vi "Display.vi"(8 "error in":errorcluster, 11 "Timeout One Button in":refnum<class "Custom - Timeout One Button.lvclass">) -> (0 "error out":errorcluster, 3 "Timeout One Button out":refnum<class "Custom - Timeout One Button.lvclass">)   [LabVIEW 2021, in "Pop-Up.lvlib" / "Custom - Timeout One Button.lvclass"]
doc: "This vi displays the custom image one button timeout popup.\n\n<b>Code Developed By:</b> +\nDaniel Coons +\nhttps://github.com/danielcoons/tsc-pop-up"
uses:
  Custom - Timeout One Button.lvclass
  C:/Development/Open Source/tsc-pop-up/Popup/Popup.lvclass
  Custom - Timeout One Button.lvclass/Custom - Timeout One Button.ctl
  Popup/Popup.lvclass/Popup.ctl
  Popup/Data Member Access/Read Theme.vi
  Theme/Theme.lvclass
  Popup/Popup.lvclass
  user32.dll
panel:
  out "header":bool
  out "count":string
  in  "OK":bool
  out "Message":string
  out "2D Picture":picture
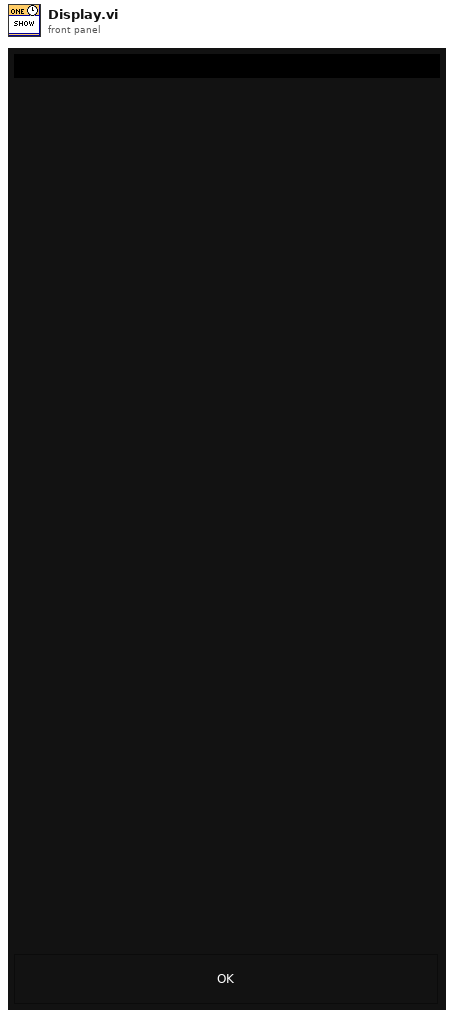
[diagram p1: front panel]
types:
  T1 = typedef "LVPoint32TypeDef.ctl" = cluster{"Horizontal":i32, "Vertical":i32}
  T2 = typedef "LVPositionTypeDef.ctl" = cluster{"Left":i32, "Top":i32}
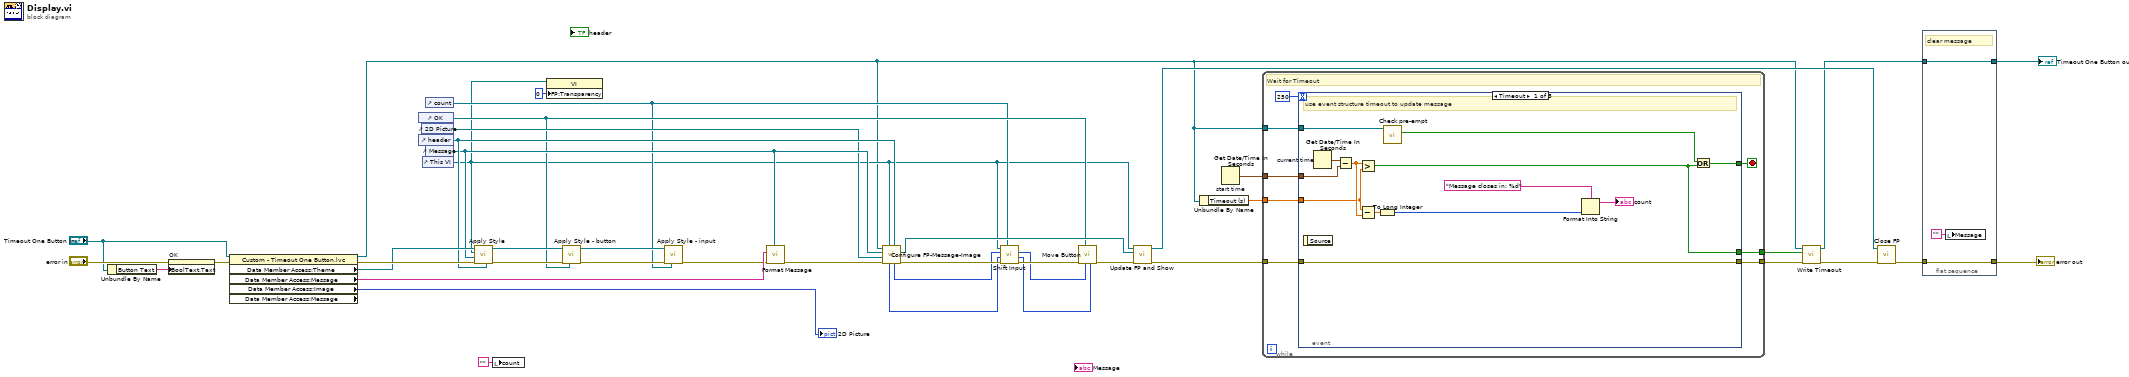
[diagram p0: block diagram]
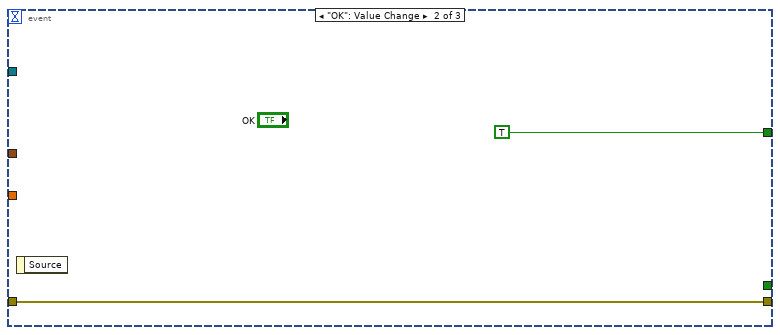
[diagram p2: hidden frame]
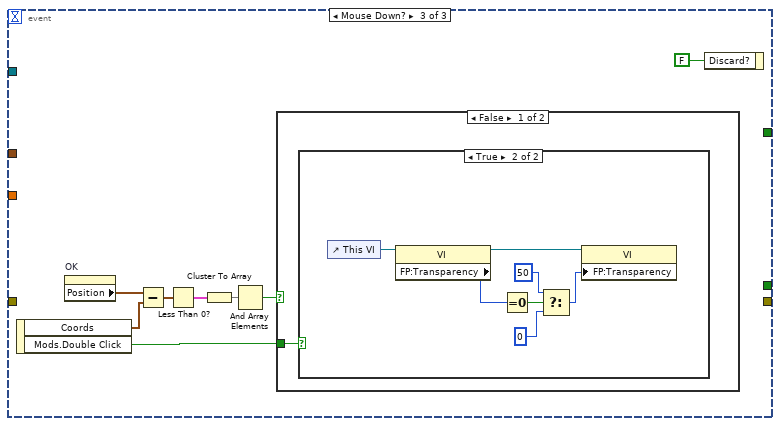
[diagram p3: hidden frame]
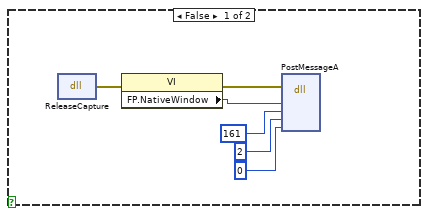
[diagram p4: hidden frame]
diagram:
  n1 = Unbundle By Name("Timeout One Button in") -> ("Button Text"=w38:string)
  n2 = property on="OK" class="Bool"(error in="error in", "BoolText.Text"=w38) -> (error out=w40:errorcluster)  [unwired: 1 in, 1 out]
  n3 = property on="Property Node" class="Custom - Timeout One Button.lvc" props=["Data Member Access:Theme", "Data Member Access:Message", "Data Member Access:Image", "Data Member Access:Message"](reference="Timeout One Button in", error in=w40) -> (reference out=w1:refnum<class "Custom - Timeout One Button.lvclass">, error out=w26:errorcluster, "Data Member Access:Theme"=w25:refnum<class "Theme.lvclass">, "Data Member Access:Message"=w23:string, "Data Member Access:Image"=→"2D Picture":picture)  [unwired: 1 out]
  n4 = control-ref of="OK"() -> (w16:refnum<vi>)
  n5 = control-ref of="header"() -> (w21:refnum<vi>)
  n6 = control-ref of="2D Picture"() -> (w19:refnum<vi>)
  n7 = control-ref of="This VI"() -> (w6:refnum<vi>)
  n8 = control-ref of="count"() -> (w11:refnum<vi>)
  n9 = control-ref of="Message"() -> (w20:refnum<vi>)
  n10 = call "Apply Style.vi"("header ref"=w21, "error in"=w26, "message ref"=w20, "pop up ref"=w6, "Theme in"=w25) -> ("error out"=w28:errorcluster, "Theme out"=w27:refnum<class "Theme.lvclass">)  [unwired: 5 in]
  n11 = local write "count"("" ("count")) -> ()
  n12 = property on="Property Node" class="VI"(reference=w6, "FP:Transparency"=u8 0 ("Front Panel Window:Transparency")) -> ()  [unwired: 1 in, 2 out]
  n13 = call "Apply Style - button.vi"("button ref"=w16, "error in"=w28, "Theme in"=w27) -> ("error out"=w24:errorcluster, "Theme out"=w13:refnum<class "Theme.lvclass">)  [unwired: 7 in]
  n14 = call "Apply Style - input.vi"("input ref"=w11, "error in (no error)"=w24, "Theme in"=w13) -> ("error out"=w14:errorcluster)  [unwired: 7 in, 1 out]
  n15 = call "Format Message.vi"("formatted string"=w20, "error in"=w14, "String Input"=w23) -> ("error out"=w22:errorcluster)  [unwired: 7 in, 1 out]
  n16 = call "Configure FP-Message-Image.vi"("header ref"=w21, "Pop Up ref"=w6, "error in (no error)"=w22, "Image ref"=w19, "Message ref"=w20, "Popup in"=w1) -> ("error out"=w18:errorcluster, "Panel Ref"=w17:refnum<vi>, "Panel Width"=w10:i32, "Panel Height"=w8:i32)  [unwired: 1 in, 1 out]
  n17 = call "Shift Input.vi"("Control"=w11, "Error In"=w18, "Panel Height"=w8, "Panel Width"=w10, "Pop Up ref"=w6) -> ("Error Out"=w12:errorcluster, "Panel Height out"=w7:i32, "Panel Width out"=w9:i32)  [unwired: 4 in]
  n18 = call "Move Button.vi"("Panel Height"=w7, "Panel Width"=w9, "Button"=w16, "error in"=w12) -> ("error out"=w15:errorcluster)  [unwired: 6 in, 1 out]
  n19 = call "Update FP and Show.vi"("error in (no error)"=w15, "Panel Ref"=w17, "VI in"=w6) -> ("error out"=w36:errorcluster, "VI out"=w32:refnum<vi>)  [unwired: 7 in]
  n20 = Unbundle By Name(w1) -> ("Timeout (s)"=w31:dbl)
  n21 = Get Date/Time In Seconds "start time"() -> (seconds since 1Jan1904=w30:timestamp)
  n22 = while {
    tunnel: [w45] -> w37
    tunnel: w36 -> [w46]
    tunnel: w30 -> [w50]
    tunnel: w31 -> [w48]
    tunnel: w1 -> [w44]
    tunnel: [w43] -> w2
    stop <- w49 stop-if-true
    # "Wait for Timeout"
    n23 = event shown="[0] Timeout" {
      selector: _ -> [_ _ _]
      dyn-events: _ -> [_ _ _]
      timeout: 250 -> [_ _ _]
      tunnel: w50 -> [w63 _ _]
      tunnel: [w54 TRUE _] -> w49
      tunnel: w48 -> [w59 _ _]
      tunnel: w46 -> [w56 w64 _]
      tunnel: [w56 w64 _] -> w45
      tunnel: w44 -> [w55 _ _]
      tunnel: [w51 _ _] -> w43
      event Timeout {
        # "use event structure timeout to update message"
        n24 = event-data() -> ()  [unwired: 1 in, 1 out]
        n25 = Get Date/Time In Seconds "current time"() -> (seconds since 1Jan1904=w62:timestamp)
        n26 = Subtract(x=w62, y=w63) -> (x-y=w61:dbl)
        n27 = Greater?(x=w61, y=w59) -> (0:w51:bool)
        n28 = Subtract(x=w59, y=w61) -> (x-y=w60:dbl)
        n29 = To Long Integer(number=w60) -> (32bit integer=w57:i32)
        n30 = call "Check pre-empt.vi"("_Popup in"=w55) -> ("Pre-empted?"=w53:bool)  [unwired: 8 in, 2 out]
        n31 = Format Into String(format string="Message closes in: %d", w57) -> (resulting string=→"count":string)  [unwired: 2 in, 1 out]
        n32 = Or(x=w53, y=w51) -> (x .or. y?=w54:bool)
      }
      event "OK": Value Change {
        n33 = event-data() -> ()  [unwired: 1 in, 1 out]
      }
      event Mouse Down? {
        n34 = event-data() -> ("Coords"=w66:T1, "Mods.Double Click"=w67:bool)  [unwired: 1 in]
        n35 = property on="OK" class="Bool"() -> ("Position"=w72:T2)  [unwired: 2 in, 2 out]
        n36 = Subtract(x=w72, y=w66) -> (x-y=w71:T2)
        n37 = Less Than 0?(x=w71) -> (x < 0?=w70:cluster{"Left":bool, "Top":bool})
        n38 = Cluster To Array(cluster=w70) -> (array=w69:bool[])
        n39 = And Array Elements(Boolean array=w69) -> (logical AND=w68:bool)
        n40 = case shown="False" w68 {
          tunnel: w67 -> [w74 _]
          frame False {
            n41 = case shown="True" w74 {
              frame False {
                n42 = dll-call lib="user32.dll" fn="ReleaseCapture"() -> (error out=w78:errorcluster)  [unwired: 4 in, 1 out]
                n43 = property on="Property Node" class="VI"(error in=w78) -> (error out=w79:errorcluster, "FP.NativeWindow"=w80:u64)  [unwired: 1 in, 1 out]
                n44 = dll-call lib="user32.dll" fn="PostMessageA"(error in=w79, "hWnd"=w80, "Msg"=161, "wParam"=2, "lParam"=0) -> ()  [unwired: 7 in, 2 out]
              }
              frame True {
                n45 = control-ref of="This VI"() -> (w87:refnum<vi>)
                n46 = property on="Property Node" class="VI"(reference=w87) -> (reference out=w85:refnum<vi>, "FP:Transparency"=w86:u8)  [unwired: 1 in, 1 out]
                n47 = Equal To 0?(x=w86) -> (x = 0?=w84:bool)
                n48 = Select(t=u8 50, s=w84, f=u8 0) -> (s? t:f=w83:u8)
                n49 = property on="Property Node" class="VI"(reference=w85, "FP:Transparency"=w83) -> ()  [unwired: 1 in, 2 out]
              }
            }
          }
          frame True {
          }
        }
        n50 = event-data ("Event Filter Node")("Discard?"=FALSE) -> ()  [unwired: 1 in, 1 out]
      }
    }
  }
  n51 = call "Write Timeout.vi"("error in"=w37, "Timeout?"=w2, "Popup in"=w1) -> ("error out"=w4:errorcluster, "Popup out"=w3:refnum<class "Custom - Timeout One Button.lvclass">)  [unwired: 7 in]
  n52 = call "Close FP.vi"("error in (no error)"=w4, "VI in"=w32) -> ("error out"=w35:errorcluster)  [unwired: 9 in]
  n53 = flat-sequence {
    tunnel: w35 -> [w90]
    tunnel: [w90] -> w34
    tunnel: w3 -> [w88]
    tunnel: [w88] -> w33
    frame #0 {
      # "clear message"
      n54 = local write "Message"("" ("Message")) -> ()
    }
  }
  "error out" <- w34
  "Timeout One Button out" <- w33
